vi "Serialize.vi"(8 "error in (no error)":errorcluster, 9 "Serialize Options":T1, 10 "Anything":variant, 11 "BlueSerializer in":refnum<class "BlueSerializer.lvclass">) -> (0 "error out":errorcluster, 2 "Serialized Text":string, 3 "BlueSerializer out":refnum<class "BlueSerializer.lvclass">)   [LabVIEW 2019, in "BlueSerialization.lvlib" / "BlueSerializer.lvclass"]
doc: "Serializes any <b>BlueSerializable</b> to a string\n\nOptions:\n<b>slice objects per SetSerializeSliceClass.vi?</b>\nIf True, then the wired object will be sliced to the class layer specified in the \"SetSerializeSliceClass override. (No-op parent will not perform any slicing.)\n\n<b>serialize non-BlueSerializable objects as hex?</b>\nIf True, then non-BlueSerializable objects will be flattened as hex data using the LabVIEW \"flatten to string\" node. If false, an error will be returned when a non-BlueSerializable object is discovered"
uses:
  BlueSerializer.lvclass
  SerializeOptions.ctl
  SerializeOptionsPayload.ctl
  ClassNameCacheMap.ctl
  ClassNameObj.ctl
  BlueSerializer.lvclass/BlueSerializer.ctl
  ClearClassNameCache.vi
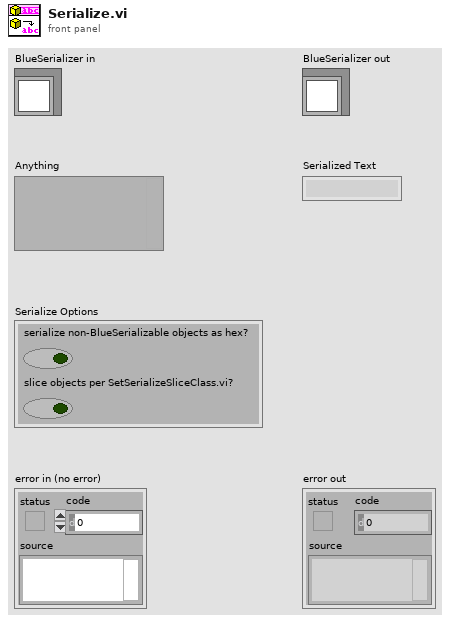
[diagram p1: front panel]
types:
  T1 = typedef "BlueSerialization.lvlib/BlueSerializer.lvclass/SerializeOptions.ctl" = cluster{"serialize non-BlueSerializable objects as hex?":bool, "slice objects per SetSerializeSliceClass.vi?":bool}
  T2 = typedef "BlueSerialization.lvlib/BlueSerializer.lvclass/SerializeOptionsPayload.ctl" = cluster{"Serialize":T1, "ClassName Cache":refnum<data-value>}
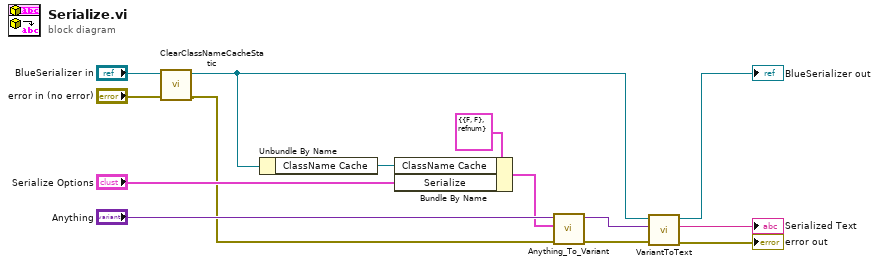
[diagram p0: block diagram]
diagram:
  n1 = call "ClearClassNameCacheStatic.vi"("error in (no error)"="error in (no error)", "BlueSerializer in"="BlueSerializer in") -> ("error out"=w3:errorcluster, "BlueSerializer out"=w2:refnum<class "BlueSerializer.lvclass">)  [unwired: 8 in]
  n2 = Unbundle By Name(w2) -> ("ClassName Cache"=w1:refnum<data-value>)
  n3 = Bundle By Name(cluster=T2 {"Serialize"={"serialize non-BlueSerializable objects as hex?"=FALSE, "slice objects per SetSerializeSliceClass.vi?"=FALSE}, "ClassName Cache"=refnum} ("Cluster"), "ClassName Cache"=w1, "Serialize"="Serialize Options") -> (w6:T2)
  n4 = call "Anything_To_Variant.vi"("error in (no error)"=w3, "Options"=w6, "Anything"="Anything") -> ("error out"=w11:errorcluster, "Serialized Variant"=w12:variant)  [unwired: 7 in]
  n5 = call-dynamic "VariantToText.vi"("error in (no error)"=w11, "Variant"=w12, "BlueSerializer in"=w2) -> ("error out"=→"error out":errorcluster, "Serializable Text"=→"Serialized Text":string, "BlueSerializer out"=→"BlueSerializer out":refnum<class "BlueSerializer.lvclass">)  [unwired: 6 in]
